vi "RSZVB Get Current Directory.vi"(8 "error in (no error)":errorcluster {"code" format="%.0x"}, 11 "VISA session":refnum<visa-resource-name>) -> (0 "error out":errorcluster {"code" format="%.0x"}, 2 "Current Directory":string, 3 "dup VISA session":refnum<visa-resource-name>)   [LabVIEW 2011]
doc: "This VI returns the default directory for mass memory storage (current directory).\n\nRemote-control command(s):\nMMEMory:CDIRectory?"
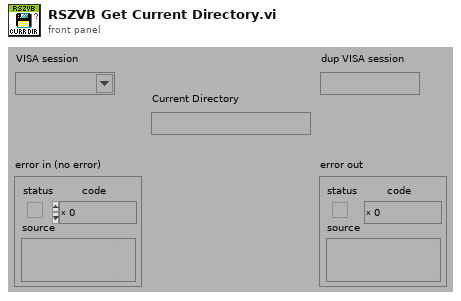
[diagram p1: front panel]
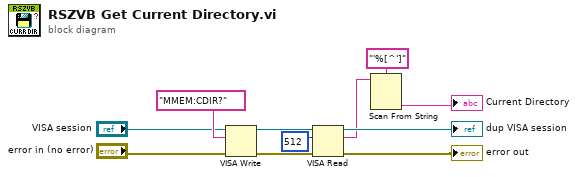
[diagram p0: block diagram]
diagram:
  n1 = VISA Write(VISA resource name="VISA session", write buffer="MMEM:CDIR?", error in (no error)="error in (no error)") -> (VISA resource name out=w10:refnum<visa-resource-name>, error out=w9:errorcluster)  [unwired: 1 out]
  n2 = VISA Read(VISA resource name=w10, byte count=u32 512 ("byte count (0)"), error in (no error)=w9) -> (VISA resource name out=→"dup VISA session":refnum<visa-resource-name>, read buffer=w2:string, error out=→"error out":errorcluster)  [unwired: 1 out]
  n3 = Scan From String(format string="'%[^']", input string=w2) -> (output 1=→"Current Directory":string)  [unwired: 3 in, 3 out]
